vi "Set Name.vi"(8 "error in":errorcluster, 10 "Name":string, 11 "Handler in":refnum<class "Handler.lvclass">) -> (0 "error out":errorcluster, 3 "Handler out":refnum<class "Handler.lvclass">)   [LabVIEW 2024, in "hse-logger.lvlib" / "Handler.lvclass"]
doc: "Sets a new ``Name`` for the handler.\n\nReturns an errror \"500009 - Invalid parameter\" if ``Name`` is empty.\n\n____\nHAMPEL SOFTWARE ENGINEERING v2.2.2 (2025-01-16 15:41)"
uses:
  <vilib>/Hampel Software Engineering/HSE Logger/Handler/Handler.lvclass
  <vilib>/Hampel Software Engineering/HSE Logger/Handler/Handler.lvclass/Handler.ctl
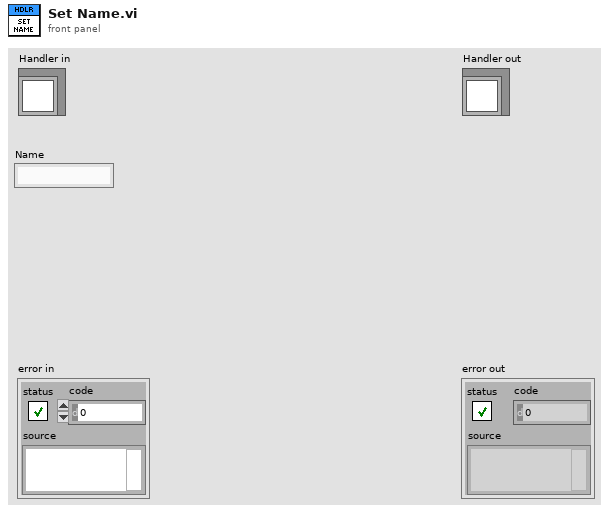
[diagram p1: front panel]
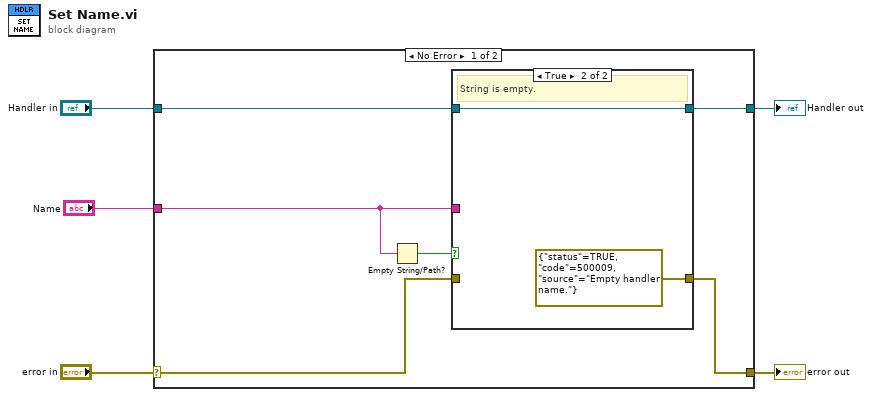
[diagram p0: block diagram]
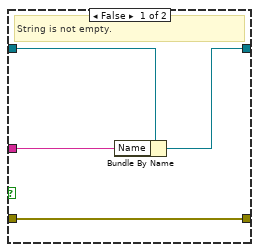
[diagram p2: hidden frame]
diagram:
  n1 = case shown="No Error" "error in" {
    selector: "error in" -> [w6 w19]
    tunnel: [w7 w19] -> w4
    tunnel: [w10 w18] -> w2
    tunnel: "Handler in" -> [w11 w18]
    tunnel: "Name" -> [w9 _]
    frame No Error {
      n2 = Empty String/Path?(string/path=w9) -> (empty?=w8:bool)
      n3 = case shown="True" w8 {
        tunnel: w11 -> [w15 w17]
        tunnel: [w14 w17] -> w10
        tunnel: w9 -> [w13 _]
        tunnel: [w12 errorcluster {"status"=TRUE, "code"=500009, "source"="Empty handler name."} ("t")] -> w7
        tunnel: w6 -> [w12 _]
        frame False {
          # "String is not empty."
          n4 = Bundle By Name(cluster=w15, "Name"=w13) -> (w14:refnum<class "Handler.lvclass">)
        }
        frame True {
          # "String is empty."
        }
      }
    }
    frame Error {
    }
  }
  "error out" <- w4
  "Handler out" <- w2
